vi "Get Input Array.vi"(8 "error in":errorcluster, 11 "Device Ref in":T1 format="%.0x") -> (0 "error out":errorcluster, 3 "Array":string[](array[string]))   [LabVIEW 2021, in "G5 Regatron Custom Device Engine.lvlib"]
uses:
  G5 Regatron Custom Device Engine.lvlib
  <vilib>/NI VeriStand/Custom Device API/Custom Device Item Ref.ctl
  <vilib>/NI VeriStand/Custom Device API/Custom Device API.lvlib
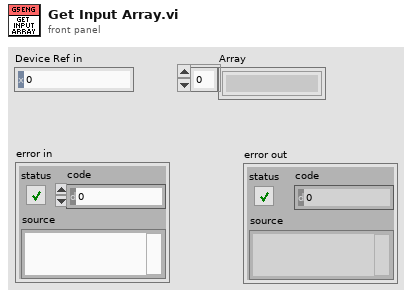
[diagram p1: front panel]
types:
  T1 = typedef "Custom Device API.lvlib/Custom Device Item Ref.ctl" = u64
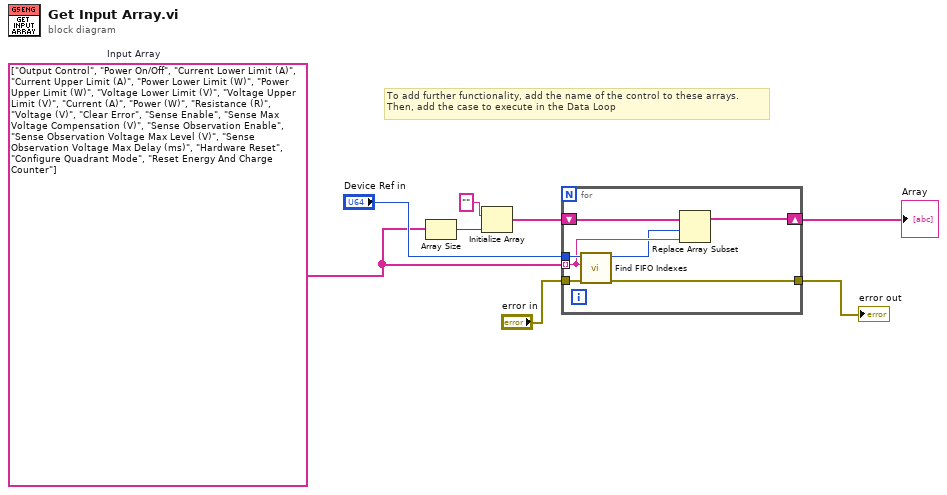
[diagram p0: block diagram]
diagram:
  w7 = string[] ["Output Control", "Power On/Off", "Current Lower Limit (A)", "Current Upper Limit (A)", "Power Lower Limit (W)", "Power Upper Limit (W)", "Voltage Lower Limit (V)", "Voltage Upper Limit (V)", "Current (A)", "Power (W)", "Resistance (R)", "Voltage (V)", "Clear Error", "Sense Enable", "Sense Max Voltage Compensation (V)", "Sense Observation Enable", "Sense Observation Voltage Max Level (V)", "Sense Observation Voltage Max Delay (ms)", "Hardware Reset", "Configure Quadrant Mode", "Reset Energy And Charge Counter"]  # Input Array
  # "To add further functionality, add the name of the control to these arrays.\nThen, add the case to execute in the Data Loop"
  n1 = Array Size(array=w7) -> (size(s)=w2:i32)
  n2 = Initialize Array("", w2) -> (w4:string[])
  n3 = for {
    tunnel: "Device Ref in" -> [w15]
    tunnel: w7 -> [w10] mode=indexing
    tunnel: "error in" -> [w14]
    tunnel: [w13] -> w6
    shift-right: [w11] -> w5
    shift-left: w4 -> [w12]
    n4 = call "Find FIFO Indexes.vi"("error in"=w14, "Item Name"=w10, "Custom Device Ref in"=w15) -> ("error out"=w13:errorcluster, "Index"=w9:i32)  [unwired: 7 in]
    n5 = Replace Array Subset(array=w12, new element=w10, index=w9) -> (w11:string[])
  }
  "error out" <- w6
  "Array" <- w5
